vi "ReportEnd_A131258.vi"(6 "文件重命名":bool, 8 "error in (no error)":errorcluster caption="错误输入（无错误）", 10 "文件名称":string, 11 "report in":refnum<class "NI_report.lvclass"> caption="报表输入") -> (0 "error out":errorcluster caption="错误输出")   [LabVIEW 2020]
uses:
  <vilib>/Utility/NIReport.llb/NI_report.lvclass
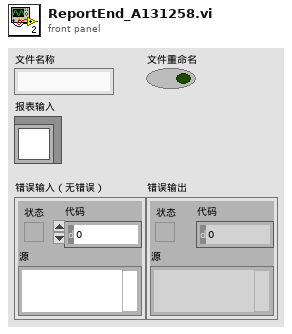
[diagram p1: front panel]
types:
  T1 = cluster{"Italic":enum16{"Italic Unchanged", "Italic On", "Italic Off"}, "Strike Through":enum16{"Strike Through Unchanged", "Strike Through On", "Strike Through Off"}, "Underline":enum16{"Underline Unchanged", "Underline On", "Underline Off"}, "Bold":enum16{"Bold Unchanged", "Bold On", "Bold Off"}}
  T2 = cluster{"Charset (-1)":i16, "Weight (-1)":i16, "Name":string, "Size":string}
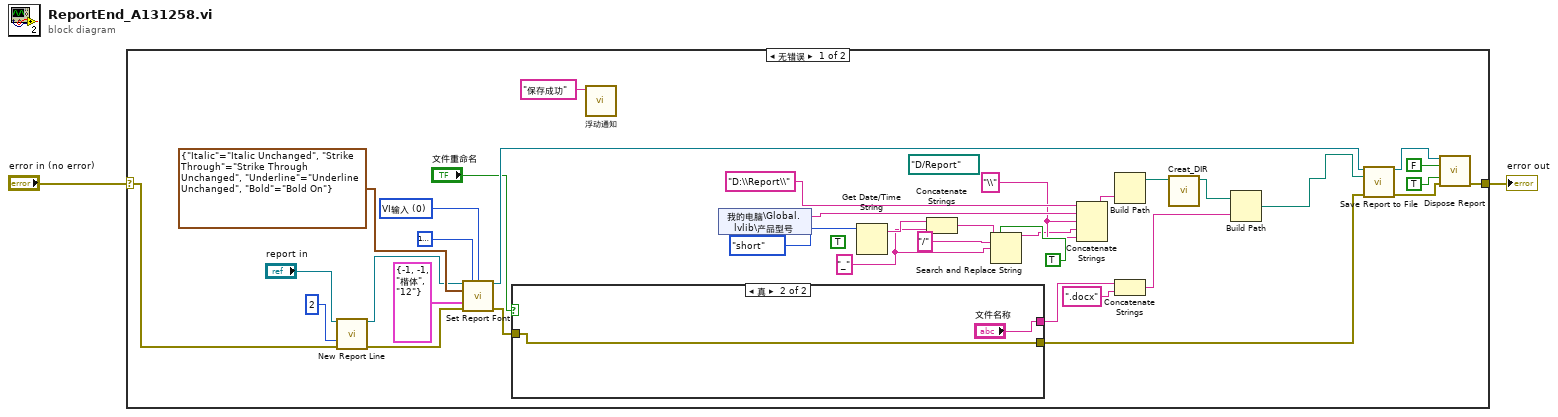
[diagram p0: block diagram]
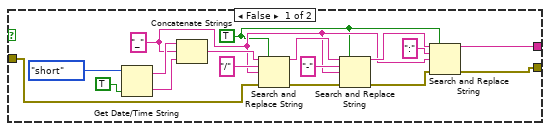
[diagram p2: hidden frame]
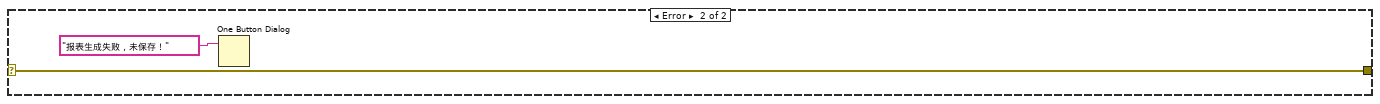
[diagram p3: hidden frame]
diagram:
  n1 = case shown="无错误" "error in (no error)" {
    selector: "error in (no error)" -> [w23 w59]
    tunnel: [w22 w59] -> w1
    frame No Error {
      w5 = "\\" ("替换字符串(\"\")")
      (unwired) TRUE ("需要秒？(F)")
      w8 = "_" ("替换字符串(\"\")")
      (unwired) path "D:/Report" ("report file path")
      w33 = u16 0 items=["VI输入", "字体对话框"] ("font settings source")
      n2 = call-dynamic "New Report Line.vi"("report in"="report in", "number of lines (1)"=2, "error in (no error)"=w23) -> ("report out"=w30:refnum<class "NI_report.lvclass">, "error out"=w29:errorcluster)  [unwired: 11 in]
      n3 = call-dynamic "Set Report Font.vi"("report in"=w30, "text color (unchanged)"=u32 16777224, "font settings source (VI Inputs)"=w33, "text options"=T1 {"Italic"=enum."Italic Unchanged", "Strike Through"=enum."Strike Through Unchanged", "Underline"=enum."Underline Unchanged", "Bold"=enum."Bold On"}, "font settings"=T2 {"Charset (-1)"=-1, "Weight (-1)"=-1, "Name"="楷体", "Size"="12"}, "error in (no error)"=w29) -> ("report out"=w26:refnum<class "NI_report.lvclass">, "error out"=w25:errorcluster)  [unwired: 7 in, 1 out]
      n4 = case shown="真" "文件重命名" {
        tunnel: [w50 "文件名称"] -> w20
        tunnel: w25 -> [w42 w56]
        tunnel: [w39 w56] -> w24
        frame False {
          w44 = TRUE ("替换全部？(F)")
          w45 = "_" ("替换字符串(\"\")")
          n5 = Get Date/Time String(date format (0)=enum16{"short", "long", "abbreviated"}."short" ("日期格式(0)"), want seconds? (F)=TRUE ("需要秒？(F)")) -> (date string=w55:string, time string=w51:string)  [unwired: 1 in]
          n6 = Concatenate Strings(w55, w45, w51) -> (w48:string)
          n7 = Search and Replace String(replace all?=w44, input string=w48, search string="/" ("搜索字符串"), replace string=w45, error in=w42) -> (result string=w47:string, error out=w41:errorcluster)  [unwired: 3 in, 2 out]
          n8 = Search and Replace String(replace all?=w44, input string=w47, search string="-" ("搜索字符串"), replace string=w45, error in=w41) -> (result string=w53:string, error out=w40:errorcluster)  [unwired: 3 in, 2 out]
          n9 = Search and Replace String(replace all?=w44, input string=w53, search string=":" ("搜索字符串"), replace string=w45, error in=w40) -> (result string=w50:string, error out=w39:errorcluster)  [unwired: 3 in, 2 out]
        }
        frame True {
        }
      }
      n10 = call "浮动通知.vi"("通知内容"="保存成功") -> ()  [unwired: 11 in]
      n11 = shared-variable "我的电脑\\Global.lvlib\\产品型号"() -> (w13:string)  [unwired: 1 in, 1 out]
      n12 = Get Date/Time String(date format (0)=enum16{"short", "long", "abbreviated"}."short" ("日期格式(0)")) -> (date string=w12:string)  [unwired: 2 in, 1 out]
      n13 = Concatenate Strings(w12, w8) -> (w11:string)
      n14 = Search and Replace String(replace all?=TRUE ("替换全部？(F)"), input string=w11, search string="/" ("搜索字符串"), replace string=w8) -> (result string=w4:string)  [unwired: 4 in, 3 out]
      n15 = Concatenate Strings("D:\\Report\\", w13, w5, w4, w5) -> (w6:string)
      n16 = Build Path(name or relative path=w6) -> (appended path=w18:path)  [unwired: 1 in]
      n17 = Concatenate Strings(w20, ".docx" ("字符串")) -> (w16:string)
      n18 = call "Creat_DIR.vi"("path"=w18) -> ("created path"=w17:path)  [unwired: 10 in]
      n19 = Build Path(base path=w17, name or relative path=w16) -> (appended path=w15:path)
      n20 = call-dynamic "Save Report to File.vi"("report in"=w26, "report file path"=w15, "error in (no error)"=w24) -> ("report out"=w38:refnum<class "NI_report.lvclass">, "error out"=w37:errorcluster)  [unwired: 11 in]
      n21 = call-dynamic "Dispose Report.vi"("report in"=w38, "wait until printing completed? (T)"=FALSE, "save changes? (F)"=TRUE, "error in (no error)"=w37) -> ("error out"=w22:errorcluster)  [unwired: 11 in]
    }
    frame Error {
      n22 = One Button Dialog(message="报表生成失败，未保存！" ("消息")) -> ()  [unwired: 1 in, 1 out]
    }
  }
  "error out" <- w1
